vi "GenerateTriggeredStimulus.vi"(8 "error in (no error)":errorcluster, 11 "Stimulus in":refnum<class "DetectSuppressionDuration.lvclass">) -> (0 "error out":errorcluster, 2 "TriggeredStimulus":sgl[][](array[numeric]), 3 "Stimulus out":refnum<class "DetectSuppressionDuration.lvclass">)   [LabVIEW 2019, in "DetectSuppressionDuration.lvclass"]
uses:
  DetectSuppressionDuration.lvclass
  DetectSuppressionDuration.lvclass/DetectSuppressionDuration.ctl
  ParametersGlobal.vi
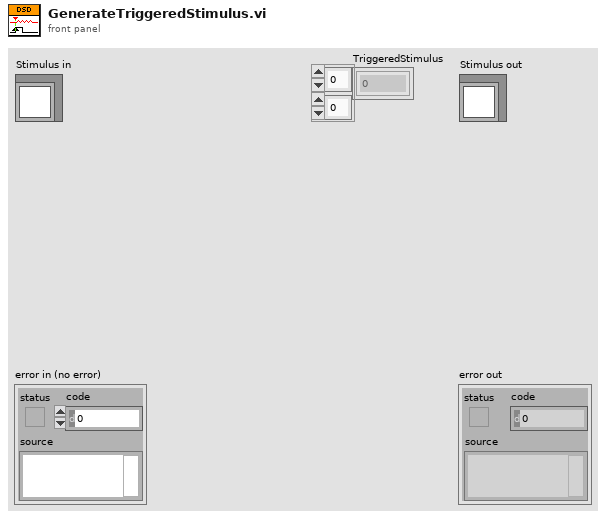
[diagram p1: front panel]
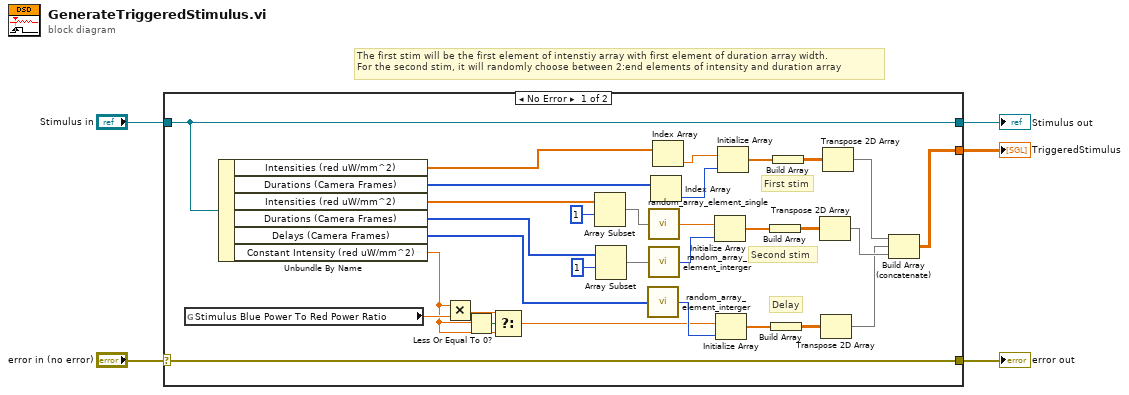
[diagram p0: block diagram]
diagram:
  # "The first stim will be the first element of intenstiy array with first element of duration array width.\nFor the second stim, it will randomly choose between 2:end elements of intensity and duration array"
  n1 = case shown="No Error" "error in (no error)" {
    selector: "error in (no error)" -> [w36 w38]
    tunnel: [w36 w38] -> w3
    tunnel: [w16 w37] -> w5
    tunnel: "Stimulus in" -> [w16 w37]
    tunnel: [w30 _] -> w4
    frame No Error {
      # "Second stim"
      # "Delay"
      # "First stim"
      n2 = global read "ParametersGlobal.vi" "Stimulus Blue Power To Red Power Ratio"() -> (w21:sgl)
      n3 = Unbundle By Name(w16) -> ("Intensities (red uW/mm^2)"=w15:sgl[], "Durations (Camera Frames)"=w13:i32[], "Intensities (red uW/mm^2)"=w9:sgl[], "Durations (Camera Frames)"=w7:i32[], "Delays (Camera Frames)"=w17:i32[], "Constant Intensity (red uW/mm^2)"=w20:sgl)
      n4 = Multiply(x=w20, y=w21) -> (x*y=w23:sgl)
      n5 = Less Or Equal To 0?(x=w20) -> (x <= 0?=w22:bool)
      n6 = Select(t=w23, s=w22, f=w20) -> (s? t:f=w19:sgl)
      n7 = Array Subset(array=w9, index=1) -> (w8:sgl[])  [unwired: 1 in]
      n8 = Array Subset(array=w7, index=1) -> (w6:i32[])  [unwired: 1 in]
      n9 = call "random_array_element_interger.vi"("Array of numbers"=w17) -> ("Randomly selected number"=w31:i32)
      n10 = call "random_array_element_single.vi"("Array of numbers"=w8) -> ("Randomly selected number"=w29:sgl)
      n11 = call "random_array_element_interger.vi"("Array of numbers"=w6) -> ("Randomly selected number"=w28:i32)
      n12 = Index Array(array=w13) -> (element=w12:i32)  [unwired: 1 in]
      n13 = Index Array(array=w15) -> (element=w14:sgl)  [unwired: 1 in]
      n14 = Initialize Array(w29, w28) -> (w27:sgl[])
      n15 = Initialize Array(w19, w31) -> (w33:sgl[])
      n16 = Initialize Array(w14, w12) -> (w35:sgl[])
      n17 = Build Array(w27) -> (w26:sgl[][])
      n18 = Build Array(w33) -> (w32:sgl[][])
      n19 = Build Array(w35) -> (w34:sgl[][])
      n20 = Transpose 2D Array(2D array=w26) -> (transposed array=w24:sgl[][])
      n21 = Transpose 2D Array(2D array=w32) -> (transposed array=w18:sgl[][])
      n22 = Transpose 2D Array(2D array=w34) -> (transposed array=w25:sgl[][])
      n23 = Build Array (concatenate)(w25, w18, w24) -> (w30:sgl[][])
    }
    frame Error {
    }
  }
  "error out" <- w3
  "Stimulus out" <- w5
  "TriggeredStimulus" <- w4
